vi "getNumberOfWheels.vi"(8 "error in (no error)":errorcluster, 11 "bus in":refnum<class "bus.lvclass">) -> (0 "error out":errorcluster, 2 "numberOfWheels":dbl, 3 "bus out":refnum<class "bus.lvclass">)   [LabVIEW 2011, in "bus.lvclass"]
uses:
  bus.lvclass
  genericVehicle.lvclass
  bus.lvclass/bus.ctl
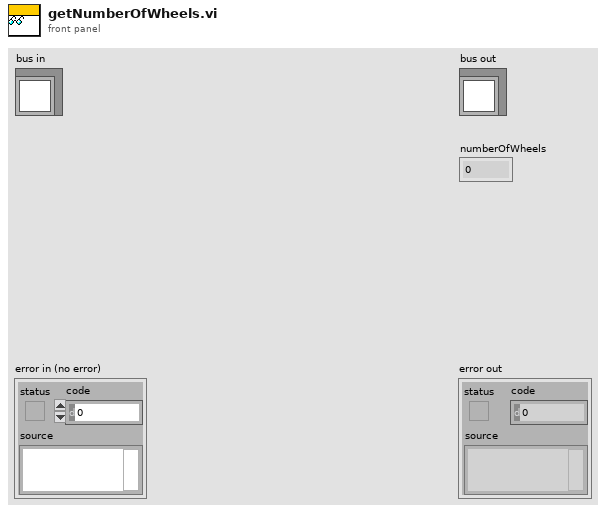
[diagram p1: front panel]
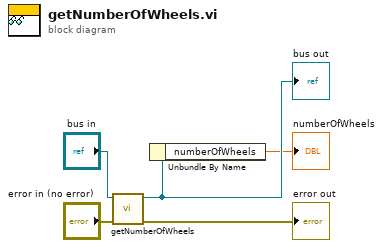
[diagram p0: block diagram]
diagram:
  n1 = call-parent "getNumberOfWheels.vi"("error in (no error)"="error in (no error)", "genericVehicle in"="bus in") -> ("error out"=→"error out":errorcluster, "genericVehicle out"=w2:refnum<class "bus.lvclass">)  [unwired: 7 in, 1 out]
  "bus out" <- w2
  n2 = Unbundle By Name(w2) -> ("numberOfWheels"=→"numberOfWheels":dbl)
